vi "WheelOfFortune Controller.vi"(8 "error in":errorcluster) -> ()   [LabVIEW 2019]
doc: "This VI executes continuously carrying out the current operation and responding to updates or new operations. It will often contain the timing or control code that is difficult to place directly in TeleOp. This VI generally opens all sensors and motors and isolates the rest of the robot code from knowing how the operations are carried out."
uses:
  WheelOfFortune Operations.ctl
  WheelOfFortune Setpoints.ctl
  <vilib>/Rock Robotics/WPI/ThirdParty/Phoenix-LabVIEW/Motor Controller/Controls/CTRE_Phoenix_MotorControl_FeedbackDevice.ctl
  <vilib>/Rock Robotics/WPI/ThirdParty/Phoenix-LabVIEW/Motor Controller/Controls/CTRE_Phoenix_MotorControl_NeutralMode.ctl
  <vilib>/Rock Robotics/WPI/ThirdParty/Phoenix-LabVIEW/Motor Controller/Controls/CTRE_Phoenix_MotorControl_ControlMode.ctl
  <vilib>/Rock Robotics/WPI/ThirdParty/Phoenix-LabVIEW/Motor Controller/Get/CTRE_Phoenix_MotorController_GetQuadratureData.vi
  <vilib>/Rock Robotics/Network Tables/NT Write Boolean.vi
  <vilib>/Rock Robotics/SystemInterfaces/i2clib/i2c_bus.ctl
panel:
  out "Matched Color Name":string
  out "Match Confidence":dbl
  out "Measured Color":cluster{"R":dbl, "G":dbl, "B":dbl}
  out "error out":errorcluster
  out "Proximity":u16(graph)
  out "Color":u32(colorbox)
  in  "Blue Calibration":cluster{"R":dbl, "G":dbl, "B":dbl}={"R"=0.143, "G"=0.427, "B"=0.429}
  in  "Green Calibration":cluster{"R":dbl, "G":dbl, "B":dbl}={"R"=0.197, "G"=0.561, "B"=0.24}
  in  "Red Calibration":cluster{"R":dbl, "G":dbl, "B":dbl}={"R"=0.561, "G"=0.323, "B"=0.114}
  in  "Yellow Calibration":cluster{"R":dbl, "G":dbl, "B":dbl}={"R"=0.361, "G"=0.524, "B"=0.113}
  in  "I2C Bus":T1
  out "Current\nCmd":string
  # "Tip: It may be helpful to observe inputs and sensor values.\nYou may also want to display tuning or debugging controls."
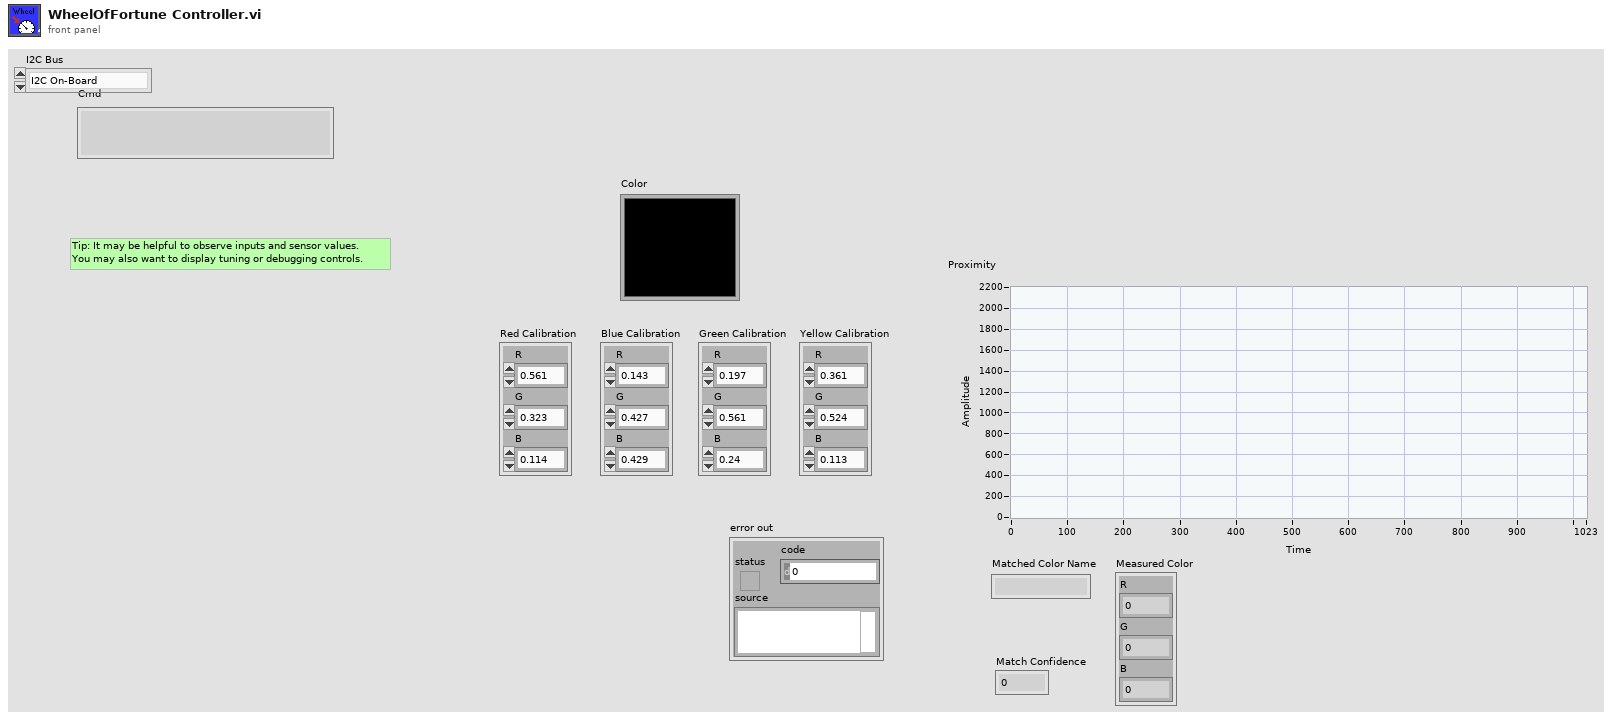
[diagram p1: front panel]
types:
  T1 = typedef "i2c_bus.ctl" = enum16{"I2C On-Board", "I2C MXP", "Invalid"}
  T2 = typedef "CTRE_Phoenix_MotorControl_ControlMode.ctl" = u16
  T3 = typedef "CTRE_Phoenix_MotorControl_NeutralMode.ctl" = enum8{"EEPROMSetting", "Override to Coast", "Override to Brake"}
  T4 = typedef "CTRE_Phoenix_MotorControl_FeedbackDevice.ctl" = i8
  T5 = typedef "WheelOfFortune Setpoints.ctl" = cluster{"Operation":T6, "Setpoint":dbl, "Duration":dbl}
  T6 = typedef "WheelOfFortune Operations.ctl" = enum16{"Reserve", "Read Current", "Immediate", "Two_Spins", "To_Color_Spin", "Up", "Down"}
  T7 = typedef "WPI_MotorControlDeviceRef.ctl" = cluster{"DeviceStatus":errorcluster, "Type":T8, "PWM":cluster{"PWM Channel":T9, "DeadBand":T10}, "CAN":cluster{"Device Number":u8, "SetOutput VI Ref":variant, "GetOutput VI Ref":variant, "Enable VI Ref":variant, "Disable VI Ref":variant, "Data":variant}, "Invert":bool, "DIO PWM":cluster{"PWM \"Enable\" Channel":T9, "DIOChannel":T11, "PWM Rate":dbl}}
  T8 = typedef "WPI_MotorControlType.ctl" = enum16{"PWM", "CAN", "DIO PWM"}
  T9 = typedef "FPGA_DIOPWMChannel.ctl" = enum8{"PWM 0", "PWM 1", "PWM 2", "PWM 3", "PWM 4", "PWM 5", "PWM 6", "PWM 7", "PWM 8", "PWM 9", "PWM MXP 0", "PWM MXP 1", "PWM MXP 2", "PWM MXP 3", "PWM MXP 4", "PWM MXP 5", "PWM MXP 6", "PWM MXP 7", "PWM MXP 8", "PWM MXP 9", "Invalid"}
  T10 = typedef "WPI_PWMDeadband.ctl" = cluster{"Name":string, "maxPositivePwm":i32, "minPositivePwm":i32, "centerPwm":i32, "maxNegativePwm":i32, "minNegativePwm":i32, "angularRange":u16}
  T11 = typedef "FPGA_DIOChannel.ctl" = enum8{"DIO 0", "DIO 1", "DIO 2", "DIO 3", "DIO 4", "DIO 5", "DIO 6", "DIO 7", "DIO 8", "DIO 9", "DIO MXP 0", "DIO MXP 1", "DIO MXP 2", "DIO MXP 3", "DIO MXP 4", "DIO MXP 5", "DIO MXP 6", "DIO MXP 7", "DIO MXP 8", "DIO MXP 9", "DIO MXP 10", "DIO MXP 11", "DIO MXP 12", "DIO MXP 13", "DIO MXP 14", "DIO MXP 15", "SPI Port CS1", "SPI Port CS2", "SPI Port CS3", "SPI Port MISO", "SPI Port MOSI", "Invalid"}
  T12 = typedef "Color Sensor V3 DevRef.ctl" = cluster{"I2CDevRef":T13}
  T13 = typedef "WPI_I2CDevRef.ctl" = cluster{"DevStatus":errorcluster, "Device Address":u8, "Handle":i32, "I2C Bus":T1}
  T14 = typedef "Command Status Info.ctl" = cluster{"Name":string, "Status":T15, "notifier out":T16}
  T15 = typedef "Completion Status.ctl" = enum16{"Successful", "Aborted", "Incomplete"}
  T16 = typedef "Completion Notifier.ctl" = refnum<notifier>
  T17 = cluster{"Current Command":T5, "Command Timing":cluster{"Start Time (ms)":u32, "Iterations":i32}, "Command Arguments":cluster{"Command Info":T14, "Description":string, "Default Command":T5, "queue out":refnum<queue>, "Subsystem Name":string}}
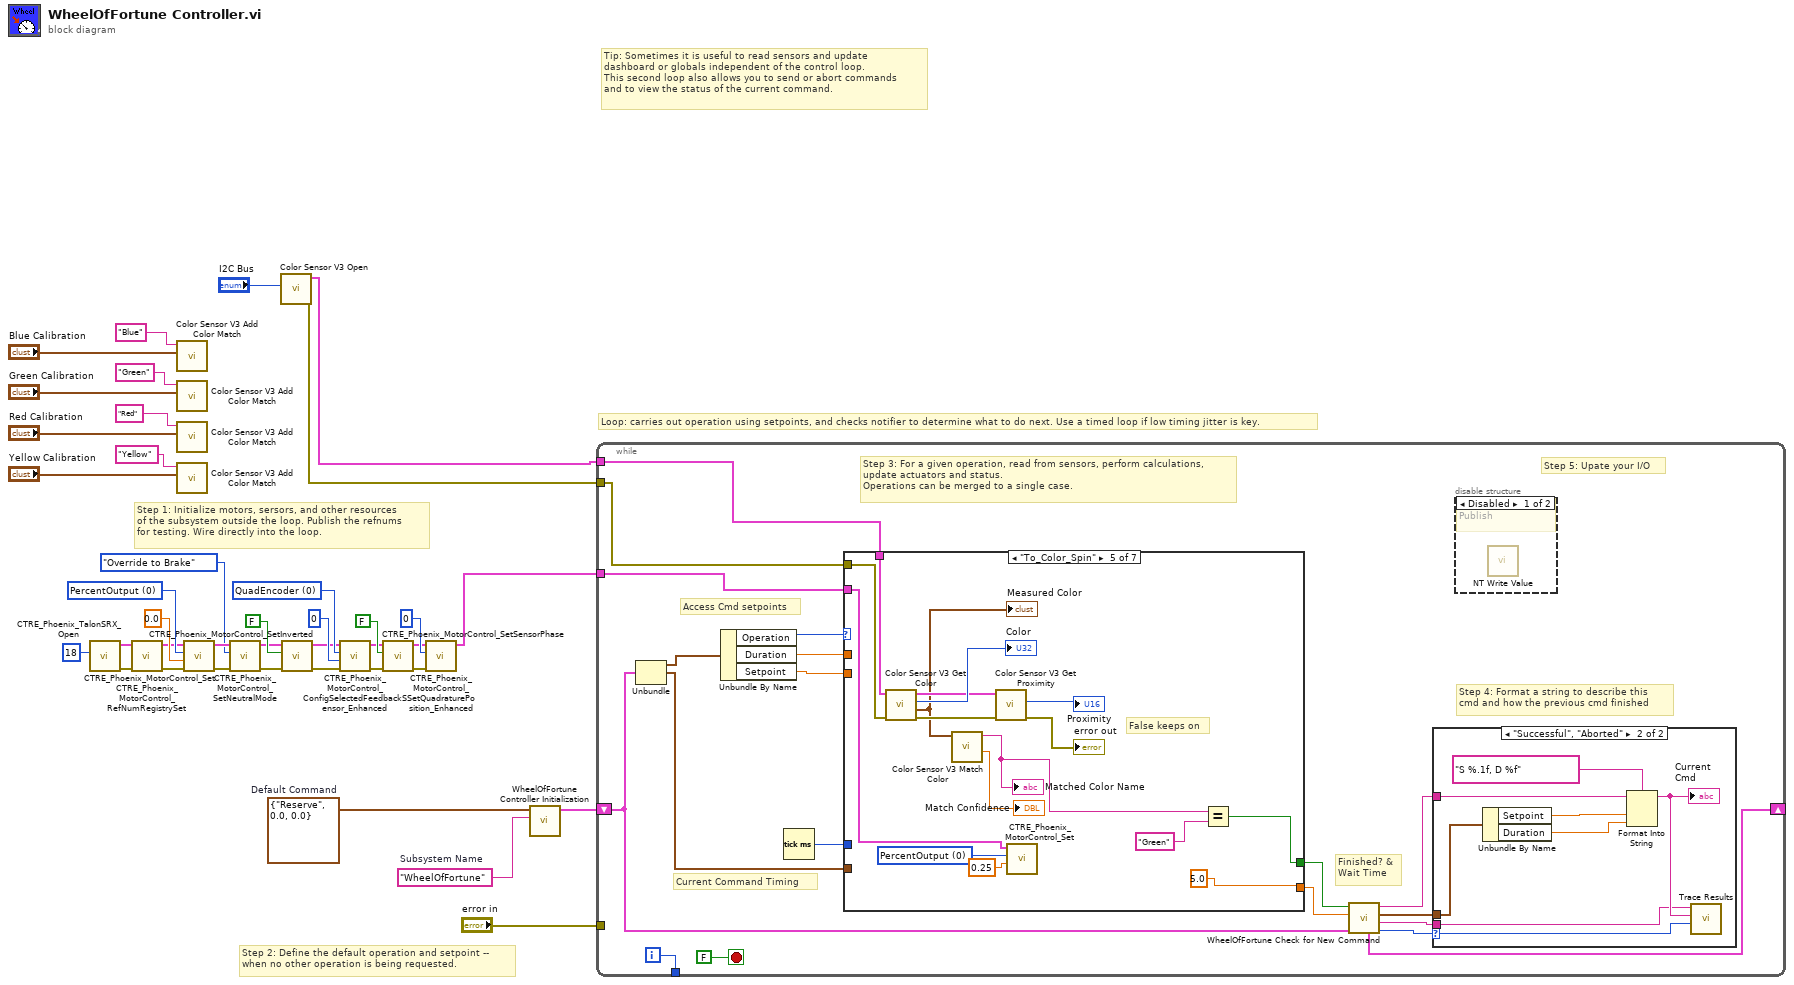
[diagram p0: block diagram]
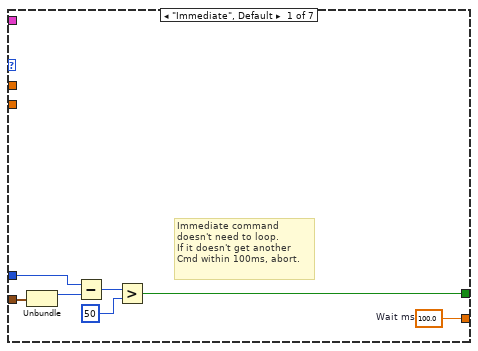
[diagram p4: hidden frame]
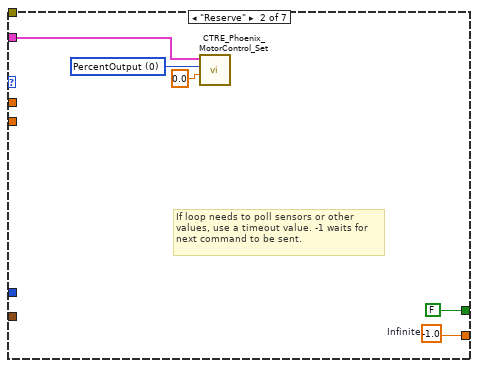
[diagram p5: hidden frame]
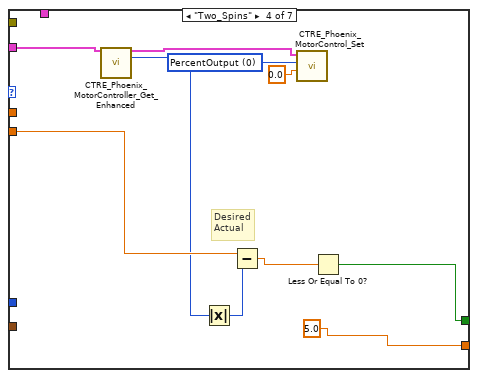
[diagram p7: hidden frame]
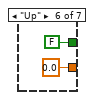
[diagram p8: hidden frame]
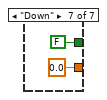
[diagram p9: hidden frame]
diagram:
  w20 = T2 0 items=["PercentOutput"=0, "Position"=1, "Velocity"=2, "Current"=3, "Follower"=5, "MotionProfile"=6, "MotionMagic"=7, "MotionProfileArc"=10, "Disabled"=15] ("Control Mode")
  w33 = T4 0 items=["QuadEncoder"=0, "Analog"=2, "Tachometer"=4, "Pulse Width Encoded Position"=8, "Sensor Sum (S0 + S1)"=9, "Sensor Difference (D0 - D1)"=10, "Remote Source 0"=11, "Remote Source 1"=12, "Software Emulated"=15] ("Feedback Device")
  w36 = T5 {"Operation"=enum."Reserve", "Setpoint"=0.0, "Duration"=0.0}  # Default Command
  w37 = "WheelOfFortune"  # Subsystem Name
  # "Tip: Sometimes it is useful to read sensors and update\ndashboard or globals independent of the control loop.\nThis second loop also allows you to send or abort commands\nand to view the status of the current command."
  # "Step 2: Define the default operation and setpoint --\nwhen no other operation is being requested."
  # "Step 1: Initialize motors, sersors, and other resources\nof the subsystem outside the loop. Publish the refnums\nfor testing. Wire directly into the loop."
  # "Loop: carries out operation using setpoints, and checks notifier to determine what to do next. Use a timed loop if low timing jitter is key."
  n1 = call <vilib>:"CTRE_Phoenix_TalonSRX_Open.vi"("Device Number"=u8 18) -> ("error out"=w35:errorcluster, "CAN Talon SRX Ref"=w34:T7)  [unwired: 9 in]
  n2 = call <vilib>:"CTRE_Phoenix_MotorControl_RefNumRegistrySet.vi"("error in (no error)"=w35, "PhoenixMotorControlDevRef"=w34) -> ("error out"=w17:errorcluster, "PhoenixMotorControlDevRef"=w18:T7)  [unwired: 8 in]
  n3 = call <vilib>:"Color Sensor V3 Add Color Match.vi"("Color"="Blue Calibration", "Name"="Blue") -> ()  [unwired: 10 in]
  n4 = call <vilib>:"Color Sensor V3 Add Color Match.vi"("Color"="Green Calibration", "Name"="Green") -> ()  [unwired: 10 in]
  n5 = call <vilib>:"Color Sensor V3 Add Color Match.vi"("Color"="Red Calibration", "Name"="Red") -> ()  [unwired: 10 in]
  n6 = call <vilib>:"Color Sensor V3 Add Color Match.vi"("Color"="Yellow Calibration", "Name"="Yellow") -> ()  [unwired: 10 in]
  n7 = call <vilib>:"CTRE_Phoenix_MotorControl_Set.vi"("error in (no error)"=w17, "Output"=0.0, "Control Mode"=w20, "PhoenixMotorControlDevRef"=w18) -> ("error out"=w16:errorcluster, "PhoenixMotorControlDevRef"=w22:T7)  [unwired: 6 in]
  n8 = call <vilib>:"CTRE_Phoenix_MotorControl_SetNeutralMode.vi"("error in (no error)"=w16, "Motor Control Neutral Mode"=CTRE_Phoenix_MotorControl_NeutralMode."Override to Brake", "PhoenixMotorControlDevRef"=w22) -> ("error out"=w15:errorcluster, "PhoenixMotorControlDevRef"=w23:T7)  [unwired: 7 in]
  n9 = call <vilib>:"Color Sensor V3 Open.vi"("I2C Bus"="I2C Bus") -> ("error out"=w1:errorcluster, "ColorSensorDevRef"=w2:T12)  [unwired: 9 in]
  n10 = call <vilib>:"CTRE_Phoenix_MotorControl_SetInverted.vi"("error in (no error)"=w15, "Invert?"=FALSE, "PhoenixMotorControlDevRef"=w23) -> ("error out"=w14:errorcluster, "PhoenixMotorControlDevRef"=w24:T7)  [unwired: 7 in]
  n11 = call <vilib>:"CTRE_Phoenix_MotorControl_ConfigSelectedFeedbackSensor_Enhanced.vi"("error in (no error)"=w14, "pidLoopIdx"=0, "Feedback Device"=w33, "PhoenixMotorControlDevRef"=w24) -> ("error out"=w26:errorcluster, "PhoenixMotorControlDevRef"=w28:T7)  [unwired: 6 in]
  n12 = call <vilib>:"CTRE_Phoenix_MotorControl_SetSensorPhase.vi"("error in (no error)"=w26, "PhaseSensor"=FALSE, "PhoenixMotorControlDevRef"=w28) -> ("error out"=w27:errorcluster, "PhoenixMotorControlDevRef"=w29:T7)  [unwired: 7 in]
  n13 = call <vilib>:"CTRE_Phoenix_MotorControl_SetQuadraturePosition_Enhanced.vi"("error in (no error)"=w27, "New Position"=0, "PhoenixMotorControlDevRef"=w29) -> ("PhoenixMotorControlDevRef"=w12:T7)  [unwired: 7 in, 1 out]
  n14 = call "WheelOfFortune Controller Initialization.vi"("Subsystem Name"=w37, "Default Command"=w36) -> ("Current Command"=w38:T17)  [unwired: 9 in]
  n15 = while {
    shift-right: [w50] -> _
    shift-left: w38 -> [w43]
    tunnel: [w57] -> _
    tunnel: "error in" -> [_]
    tunnel: w12 -> [w42]
    tunnel: w2 -> [w41]
    tunnel: w1 -> [w40]
    i -> [w57]
    stop <- FALSE stop-if-true
    # "Step 5: Upate your I/O"
    # "Step 4: Format a string to describe this\ncmd and how the previous cmd finished"
    # "Current Command Timing"
    # "Access Cmd setpoints"
    # "Finished? &\nWait Time"
    # "Step 3: For a given operation, read from sensors, perform calculations,\nupdate actuators and status.\nOperations can be merged to a single case."
    n16 = Unbundle(w43) -> ("Current Command"=w56:T5, "Command Timing"=w52:cluster{"Start Time (ms)":u32, "Iterations":i32})  [unwired: 1 out]
    n17 = Unbundle By Name(w56) -> ("Operation"=w55:T6, "Duration"=w54:dbl, "Setpoint"=w51:dbl)
    n18 = Tick Count (ms)() -> (millisecond timer value=w53:u32)
    n19 = case shown="\"To_Color_Spin\"" w55 {
      tunnel: [w73 w78 _ 5.0 ("y") 5.0 ("y") 0.0 ("y") 0.0 ("y")] -> w48
      tunnel: [w67 FALSE ("ignore previous (F)") _ w85 w91 FALSE ("ignore previous (F)") FALSE ("ignore previous (F)")] -> w49
      tunnel: w52 -> [w69 _ _ _ _ _ _]
      tunnel: w54 -> [_ _ _ _ _ _ _]
      tunnel: w53 -> [w68 _ _ _ _ _ _]
      tunnel: w51 -> [_ _ _ w84 _ _ _]
      tunnel: w42 -> [_ w76 _ w82 w92 _ _]
      tunnel: w41 -> [_ _ _ _ w96 _ _]
      tunnel: w40 -> [_ _ _ _ w95 _ _]
      frame "Immediate", Default {
        w73 = 100.0  # Wait ms
        # "Immediate command\ndoesn't need to loop.\nIf it doesn't get another\nCmd within 100ms, abort."
        n20 = Unbundle(w69) -> ("Start Time (ms)"=w72:u32)  [unwired: 1 out]
        n21 = Subtract(x=w68, y=w72) -> (x-y=w71:u32)
        n22 = Greater?(x=w71, y=u8 50 ("Left Motor")) -> (0:w67:bool)
      }
      frame "Reserve" {
        w74 = T2 0 items=["PercentOutput"=0, "Position"=1, "Velocity"=2, "Current"=3, "Follower"=5, "MotionProfile"=6, "MotionMagic"=7, "MotionProfileArc"=10, "Disabled"=15] ("Control Mode")
        w78 = -1.0  # Infinite
        # "If loop needs to poll sensors or other\nvalues, use a timeout value. -1 waits for\nnext command to be sent."
        n23 = call <vilib>:"CTRE_Phoenix_MotorControl_Set.vi"("Output"=0.0, "Control Mode"=w74, "PhoenixMotorControlDevRef"=w76) -> ()  [unwired: 7 in, 2 out]
      }
      frame "Read Current" {
      }
      frame "Two_Spins" {
        w80 = T2 0 items=["PercentOutput"=0, "Position"=1, "Velocity"=2, "Current"=3, "Follower"=5, "MotionProfile"=6, "MotionMagic"=7, "MotionProfileArc"=10, "Disabled"=15] ("Control Mode")
        # "Desired\nActual"
        n24 = call-poly <vilib>:"CTRE_Phoenix_MotorController_Get_Enhanced.vi"("PhoenixMotorControlDevRef"=w82) -> ("PhoenixMotorControlDevRef"=w79:T7, "Quadrature Position"=w83:i32)  [unwired: 11 in, 2 out]
        n25 = Absolute Value(x=w83) -> (abs(x)=w88:i32)
        n26 = Subtract(x=w84, y=w88) -> (x-y=w87:dbl)
        n27 = call <vilib>:"CTRE_Phoenix_MotorControl_Set.vi"("Output"=0.0, "Control Mode"=w80, "PhoenixMotorControlDevRef"=w79) -> ()  [unwired: 7 in, 2 out]
        n28 = Less Or Equal To 0?(x=w87) -> (x <= 0?=w85:bool)
      }
      frame "To_Color_Spin" {
        w93 = T2 0 items=["PercentOutput"=0, "Position"=1, "Velocity"=2, "Current"=3, "Follower"=5, "MotionProfile"=6, "MotionMagic"=7, "MotionProfileArc"=10, "Disabled"=15] ("Control Mode")
        # "False keeps on"
        n29 = call <vilib>:"Color Sensor V3 Get Color.vi"("error in (no error)"=w95, "ColorSensorDevRef"=w96) -> ("error out"=w102:errorcluster, "Normalized Color"=w98:cluster{"R":dbl, "G":dbl, "B":dbl}, "Color"=→"Color":u32, "ColorSensorDevRef out"=w101:T12)  [unwired: 6 in]
        "Measured Color" <- w98
        n30 = call <vilib>:"Color Sensor V3 Match Color.vi"("Measured Color"=w98) -> ("Confidence"=→"Match Confidence":dbl, "Matched Color Name"=w90:string)  [unwired: 8 in, 1 out]
        "Matched Color Name" <- w90
        n31 = call <vilib>:"Color Sensor V3 Get Proximity.vi"("error in (no error)"=w102, "ColorSensorDevRef"=w101) -> ("error out"=→"error out":errorcluster, "Proximity"=→"Proximity":u16)  [unwired: 7 in, 1 out]
        n32 = call <vilib>:"CTRE_Phoenix_MotorControl_Set.vi"("Output"=0.25, "Control Mode"=w93, "PhoenixMotorControlDevRef"=w92) -> ()  [unwired: 7 in, 2 out]
        n33 = Equal?(x=w90, y="Green") -> (x = y?=w91:bool)
      }
      frame "Up" {
      }
      frame "Down" {
      }
    }
    n34 = call "WheelOfFortune Check for New Command.vi"("Current Command"=w43, "Wait time (ms)"=w48, "Finished?"=w49) -> ("Completion"=w44:T15, "Subsystem Name"=w45:string, "Current Command"=w46:T5, "Initial Trace String"=w47:string, "NextCommand"=w50:T17)  [unwired: 4 in]
    n35 = case shown="\"Successful\", \"Aborted\"" w44 {
      selector: w44 -> [_ w66]
      tunnel: w47 -> [_ w62]
      tunnel: w46 -> [_ w63]
      tunnel: w45 -> [_ w59]
      frame "Incomplete", Default {
        # "Continuing current command"
      }
      frame "Successful", "Aborted" {
        # "Report and setup for next command"
        n36 = Unbundle By Name(w63) -> ("Setpoint"=w65:dbl, "Duration"=w60:dbl)
        n37 = Format Into String(format string="S %.1f, D %f", initial string=w62, w65, w60) -> (resulting string=w61:string)  [unwired: 1 in, 1 out]
        "Current\nCmd" <- w61
        n38 = call <vilib>:"Trace Results.vi"("Status of previous command"=w66, "Description"=w61, "Subsystem"=w59) -> ()  [unwired: 9 in]
      }
    }
    n39 = disable-structure shown="Disabled" {
      frame Disabled {
        # "Publish"
        n40 = call-poly <vilib>:"NT Write Value.vi"() -> ()  [unwired: 11 in, 1 out]
      }
      frame Enabled {
      }
    }
  }
